vi "CSM - Read Cluster Elements From Key.vi"(5 "Section Name(\"\" as Default)":string, 8 "error in (no error)":errorcluster, 9 "Cluster":variant) -> (2 "error out":errorcluster, 3 "Cluster out":variant)   [LabVIEW 2017, in "INI-Static-Variable-Support.lvlib"]
uses:
  INI-Static-Variable-Support.lvlib
  <userlib>/_NEVSTOP/Communicable State Machine(CSM)/addons/API-String-Arugments-Support/API String Arguments Support.lvlib
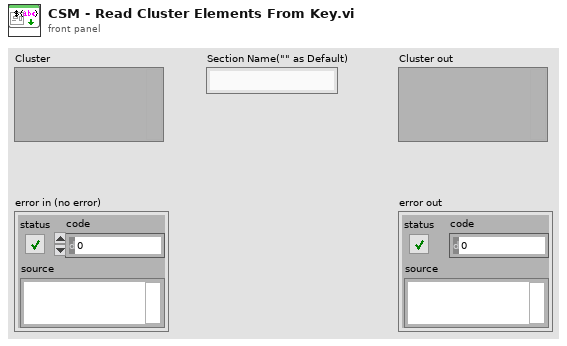
[diagram p1: front panel]
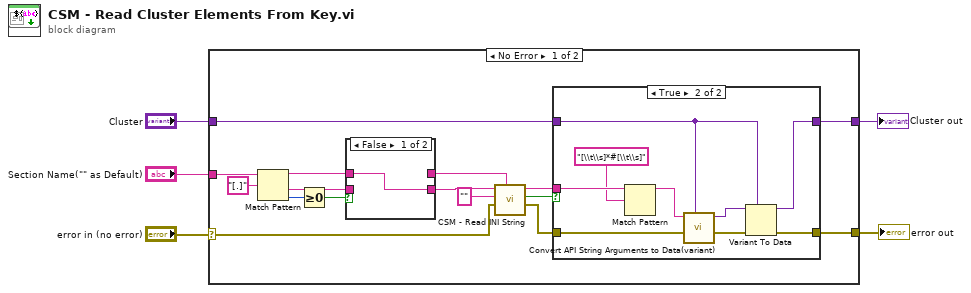
[diagram p0: block diagram]
diagram:
  n1 = case shown="No Error" "error in (no error)" {
    selector: "error in (no error)" -> [w12 w36]
    tunnel: [w6 w36] -> w5
    tunnel: "Section Name(\"\" as Default)" -> [w21 _]
    tunnel: "Cluster" -> [w9 w37]
    tunnel: [w10 w37] -> w1
    frame No Error {
      n2 = Match Pattern(string=w21, regular expression="[.]") -> (before substring=w17:string, after substring=w16:string, offset past match=w19:i32)  [unwired: 1 in, 1 out]
      n3 = Greater Or Equal To 0?(x=w19) -> (x >= 0?=w18:bool)
      n4 = case shown="False" w18 {
        tunnel: w17 -> [w22 w23]
        tunnel: w16 -> [_ w24]
        tunnel: [w22 w24] -> w14
        tunnel: [_ w23] -> w15
        frame False {
        }
        frame True {
        }
      }
      n5 = call "CSM - Read INI String.vi"("Section Name(\"\" as Default)"=w15, "error in (no error)"=w12, ">> Default Value >>"="", "String in"=w14) -> ("error out"=w7:errorcluster, "Key Found?"=w11:bool, "String out"=w8:string)  [unwired: 3 in]
      n6 = case shown="True" w11 {
        tunnel: [w26 w33] -> w10
        tunnel: w9 -> [w26 w31]
        tunnel: w8 -> [_ w35]
        tunnel: w7 -> [w25 w27]
        tunnel: [w25 w28] -> w6
        frame False {
        }
        frame True {
          n7 = Match Pattern(string=w35, regular expression="[\\t\\s]*#[\\t\\s]") -> (before substring=w30:string)  [unwired: 1 in, 3 out]
          n8 = call <userlib>:"Convert API String Arguments to Data(variant).vi"("Type"=w31, "error in (no error)"=w27, "String"=w30) -> ("error"=w29:errorcluster, "Data"=w32:variant)  [unwired: 7 in]
          n9 = Variant To Data(error in=w29, type=w31, Variant=w32) -> (data=w33:variant, error out=w28:errorcluster)
        }
      }
    }
    frame Error {
    }
  }
  "error out" <- w5
  "Cluster out" <- w1
